vi "GetStringControl.vi"(8 "error in (no error)":errorcluster, 10 "Name":string, 11 "VIEW in":refnum<class "VIEW.lvclass">) -> (0 "error out":errorcluster, 2 "Text.Text":string, 3 "VIEW out":refnum<class "VIEW.lvclass">)   [LabVIEW 2013, in "VIEW.lvclass"]
uses:
  VIEW.lvclass
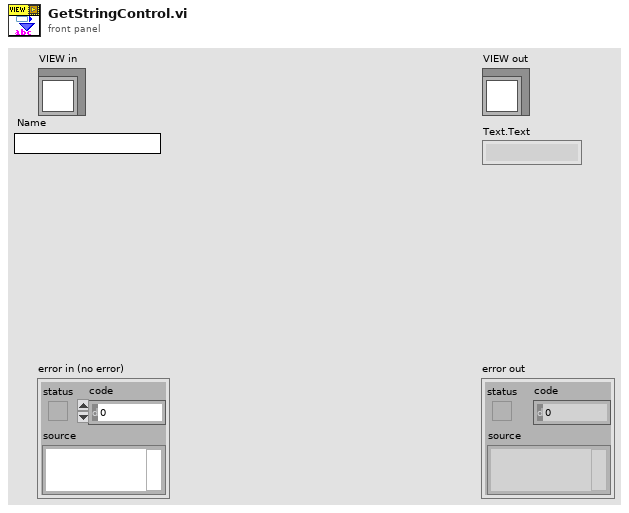
[diagram p1: front panel]
types:
  T1 = cluster{"CtlRef":refnum<vi>, "Name":string, "ClassName":string}
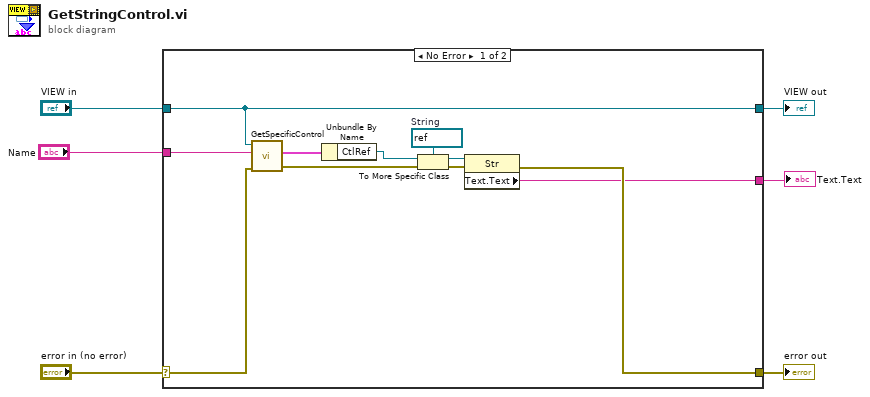
[diagram p0: block diagram]
diagram:
  n1 = case shown="No Error" "error in (no error)" {
    selector: "error in (no error)" -> [w9 w19]
    tunnel: [w8 w19] -> w5
    tunnel: [w17 w18] -> w3
    tunnel: "VIEW in" -> [w17 w18]
    tunnel: "Name" -> [w16 _]
    tunnel: [w7 _] -> w1
    frame No Error {
      w13 = refnum<vi> refnum  # String
      n2 = call "GetSpecificControl.vi"("error in (no error)"=w9, "Name"=w16, "VIEW in"=w17) -> ("error out"=w10:errorcluster, "output cluster"=w11:T1)  [unwired: 6 in, 1 out]
      n3 = Unbundle By Name(w11) -> ("CtlRef"=w12:refnum<vi>)
      n4 = To More Specific Class(target class=w13, reference=w12, error in=w10) -> (specific class reference=w14:refnum<vi>, error out=w15:errorcluster)
      n5 = property class="Str"(reference=w14, error in=w15) -> (error out=w8:errorcluster, "Text.Text"=w7:string)  [unwired: 1 out]
    }
    frame Error {
    }
  }
  "error out" <- w5
  "VIEW out" <- w3
  "Text.Text" <- w1
